vi "Test Sweep Manager.vi"(8 "error in (no error)":errorcluster, 11 "Generator in":refnum<class "Generator.lvclass">) -> (0 "error out":errorcluster, 3 "Generator out":refnum<class "Generator.lvclass">)   [LabVIEW 2019, in "Generator.lvclass"]
uses:
  Generator.lvclass
  typedefs/Sampling--Cluster.ctl
  typedefs/Sweep.Configuration--Cluster.ctl
  typedefs/Sweep.Channel--Cluster--Array.ctl
  typedefs/Sweep.Channel--Cluster.ctl
  typedefs/Sweep.Pattern--Enum.ctl
  typedefs/AO.Channel--Cluster--Array.ctl
  typedefs/AO.Channel--Cluster.ctl
  typedefs/AO.Channel.Function--Enum.ctl
  Generator.lvclass/Generator.ctl
  typedefs/Generator.Sweep Status--enum.ctl
  typedefs/Generator.Command--enum.ctl
  Waveform.Attributes/Waveform.Attributes.lvlib
panel:
  in  "AO Channels":T1=[{"Enable?"=TRUE, "Channel"=1, "Amplitude"=0.1, "Offset"=0.0, "Frequency"=13.0, "Phase"=0.0, "Function"=enum."sine", "Sweeping?"=FALSE, "Limit AC?"=FALSE, "Limit DC?"=FALSE, "Duty Cycle?"=FALSE, "Duty Cycle"=0.0}, {"Enable?"=TRUE, "Channel"=0, "Amplitude"=0.0, "Offset"=0.09, "Frequency"=0.1, "Phase"=0.0, "Function"=enum."sine", "Sweeping?"=FALSE, "Limit AC?"=FALSE, "Limit DC?"=FALSE, "Duty Cycle?"=FALSE, "Duty Cycle"=0.0}, {"Enable?"=TRUE, "Channel"=0, "Amplitude"=0.0, "Offset"=0.0, "Frequency"=0.1, "Phase"=0.0, "Function"=enum."sine", "Sweeping?"=FALSE, "Limit AC?"=FALSE, "Limit DC?"=FALSE, "Duty Cycle?"=FALSE, "Duty Cycle"=0.0}, {"Enable?"=TRUE, "Channel"=0, "Amplitude"=0.0, "Offset"=0.01, "Frequency"=0.1, "Phase"=0.0, "Function"=enum."sine", "Sweeping?"=FALSE, "Limit AC?"=FALSE, "Limit DC?"=FALSE, "Duty Cycle?"=FALSE, "Duty Cycle"=0.0}]
  out "Appended vs sample":dbl[][](graph)
  out "Concatenated":waveform(dbl)[](graph)
  out "Appended vs time":waveform(dbl)[](graph)
  in  "Sweep Pattern":cluster{"Channel":u16, "Sweep Pattern":dbl[]}[](array[cluster])=[{"Channel"=4, "Sweep Pattern"=[0.01, 0.02, 0.015, 0.025, 0.02, 0.03]}] {"Sweep Pattern" format="%#_3p"; "Channel" min=1 max=128}
  out "Updates":i32=14
  out "Live":waveform(dbl)[](graph)
  in  "Configuration.Sweep":T4={"Sweep Time (s)"=100.0, "Initial Wait (s)"=0.1, "Return to Start"=TRUE, "Channels"=[{"Enable?"=TRUE, "Channel"=1, "Start"=0.0, "End"=0.1, "Pattern"=enum."Smooth Ramp _/\\_", "Table"=[]}, {"Enable?"=TRUE, "Channel"=2, "Start"=0.09, "End"=0.09, "Pattern"=enum."Smooth Ramp _/\\_", "Table"=[]}, {"Enable?"=TRUE, "Channel"=3, "Start"=0.0, "End"=0.01, "Pattern"=enum."Ramp /\\", "Table"=[]}, {"Enable?"=TRUE, "Channel"=4, "Start"=0.01, "End"=0.011, "Pattern"=enum."Table", "Table"=[]}]} {"Channels"."Table" format="%#_1f"; "Channels"."Channel" min=1 max=128; "Channels"."Start" format="%#_6p"; "Channels"."End" format="%#_6p"}
  in  "Sampling":T8={"Fs"=10000.0, "#s"=1000.0}
  in  "stop":bool
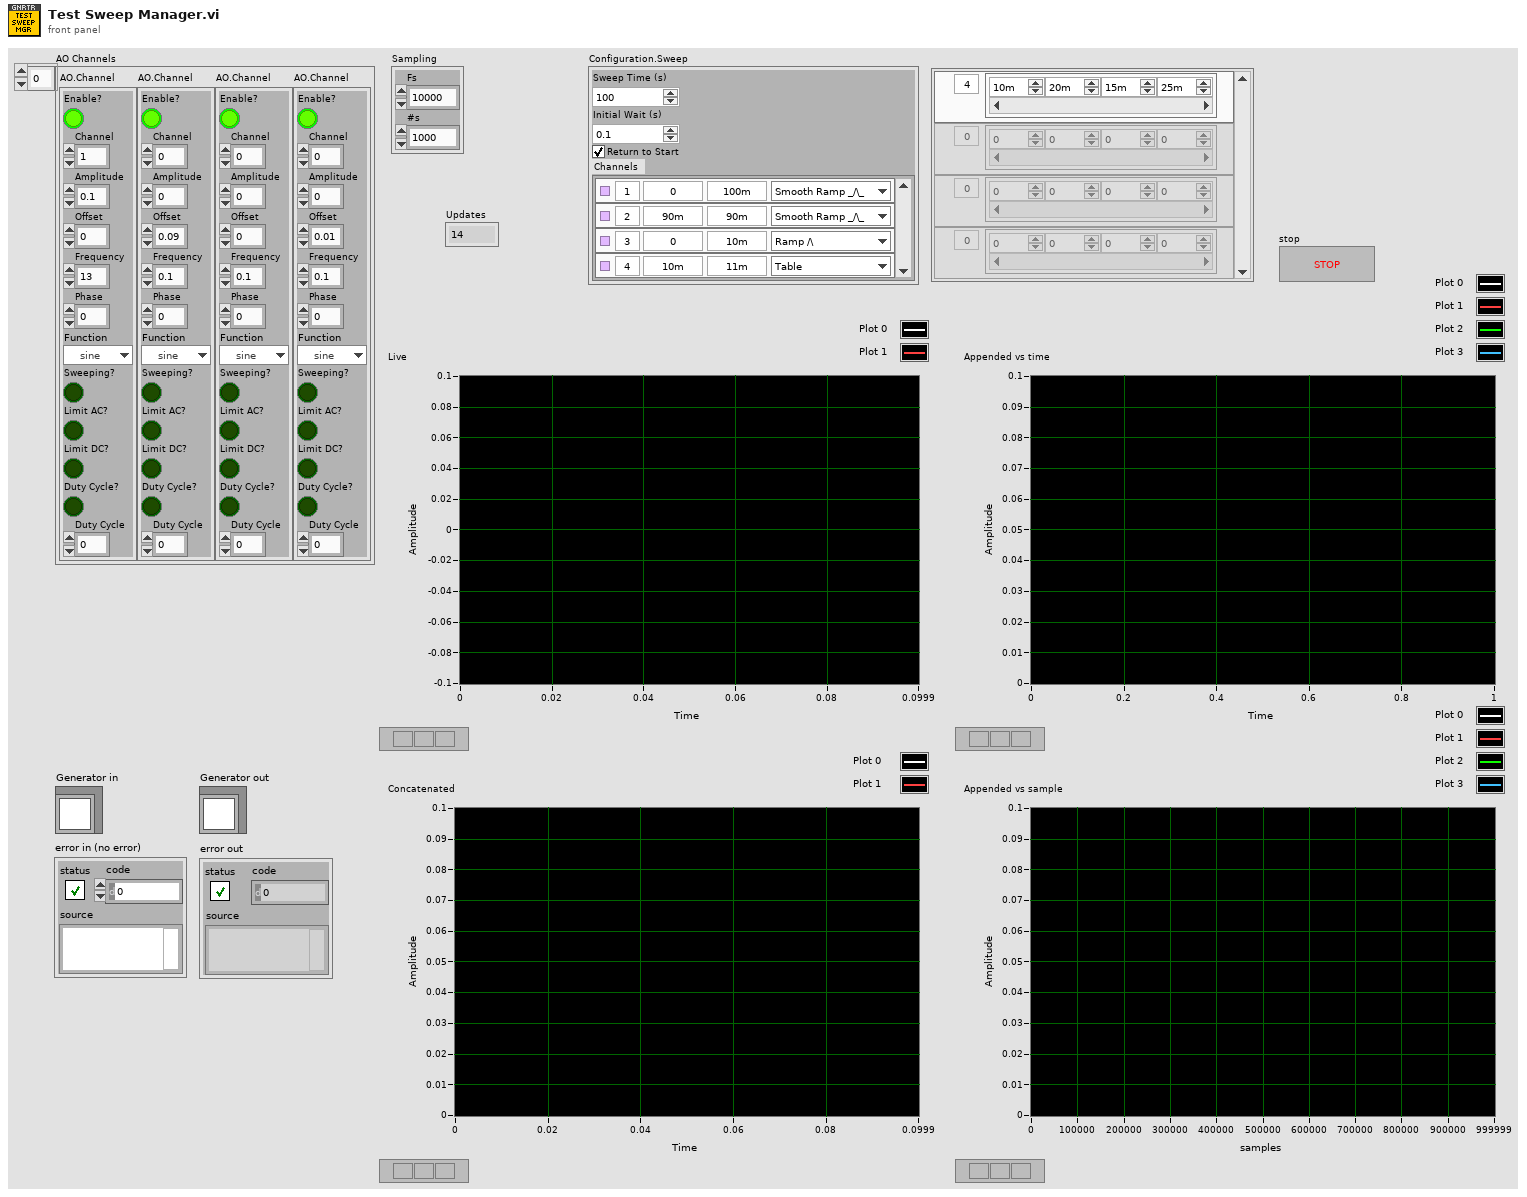
[diagram p1: front panel]
types:
  T1 = typedef "Generator.lvclass/AO.Channel--Cluster--Array.ctl" = T2[]
  T2 = typedef "Generator.lvclass/AO.Channel--Cluster.ctl" = cluster{"Enable?":bool, "Channel":i32, "Amplitude":dbl, "Offset":dbl, "Frequency":dbl, "Phase":dbl, "Function":T3, "Sweeping?":bool, "Limit AC?":bool, "Limit DC?":bool, "Duty Cycle?":bool, "Duty Cycle":dbl}
  T3 = typedef "Generator.lvclass/AO.Channel.Function--Enum.ctl" = enum16{"sine", "square", "triangle", "saw"}
  T4 = typedef "Generator.lvclass/Sweep.Configuration--Cluster.ctl" = cluster{"Sweep Time (s)":dbl, "Initial Wait (s)":dbl, "Return to Start":bool, "Channels":T5}
  T5 = typedef "Generator.lvclass/Sweep.Channel--Cluster--Array.ctl" = T6[]
  T6 = typedef "Generator.lvclass/Sweep.Channel--Cluster.ctl" = cluster{"Enable?":bool, "Channel":u16, "Start":dbl, "End":dbl, "Pattern":T7, "Table":dbl[]}
  T7 = typedef "Generator.lvclass/Sweep.Pattern--Enum.ctl" = enum16{"Ramp /", "Ramp /\\", "Smooth Ramp _/", "Smooth Ramp _/\\_", "Table"}
  T8 = typedef "Generator.lvclass/Sampling--Cluster.ctl" = cluster{"Fs":dbl, "#s":dbl}
  T9 = typedef "Generator.lvclass/Generator.Sweep Status--enum.ctl" = enum16{"idle", "initializing", "waiting", "sweeping", "stopping"}
  T10 = typedef "Generator.lvclass/Generator.Command--enum.ctl" = enum16{"start", "stop", "start sweep", "stop sweep"}
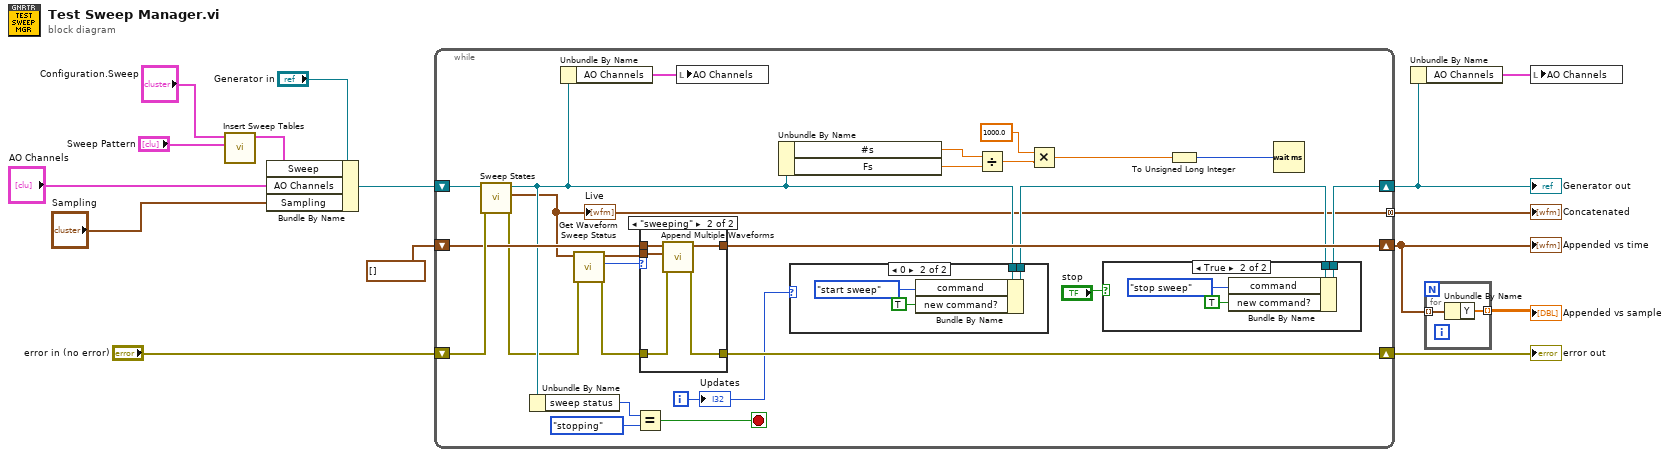
[diagram p0: block diagram]
diagram:
  n1 = call "Insert Sweep Tables.vi"("Channels New"="Sweep Pattern", "Sweep Configuration in"="Configuration.Sweep") -> ("Sweep Configuration out"=w11:T4)  [unwired: 9 in]
  n2 = Bundle By Name(cluster="Generator in", "Sweep"=w11, "AO Channels"="AO Channels", "Sampling"="Sampling") -> (w3:refnum<class "Generator.lvclass">)
  n3 = while {
    shift-right: [w39] -> w15
    shift-left: "error in (no error)" -> [w40]
    shift-right: [w35] -> w8
    shift-left: w3 -> [w36]
    shift-right: [w37] -> w2
    shift-left: waveform(dbl)[] [] ("Waveform out []") -> [w38]
    tunnel: [w20] -> w6 mode=concatenating
    i -> [w32]
    stop <- w30 stop-if-true
    n4 = call "Sweep States.vi"("error in (no error)"=w40, "Generator in"=w36) -> ("error out"=w17:errorcluster, "Waveforms out"=w20:waveform(dbl)[], "Generator out"=w29:refnum<class "Generator.lvclass">)  [unwired: 7 in]
    "Live" <- w20
    n5 = Unbundle By Name(w29) -> ("sweep status"=w21:T9)
    n6 = Unbundle By Name(w29) -> ("AO Channels"=w22:T1)
    n7 = call "Get Waveform Sweep Status.vi"("error in (no error)"=w17, "Waveforms in"=w20) -> ("error out"=w16:errorcluster, "sweep status"=w18:T9, "Waveforms out"=w19:waveform(dbl)[])  [unwired: 7 in]
    n8 = Equal?(x=w21, y=Generator.Sweep_Status--enum."stopping") -> (x = y?=w30:bool)
    n9 = case shown="\"sweeping\"" w18 {
      tunnel: [w41 w47] -> w39
      tunnel: w16 -> [w41 w46]
      tunnel: w19 -> [_ w43]
      tunnel: w38 -> [w42 w45]
      tunnel: [w42 w44] -> w37
      frame Default {
      }
      frame "sweeping" {
        n10 = call "Append Multiple Waveforms.vi"("error in (no error)"=w46, "Waveform B []"=w43, "Waveforrm A []"=w45) -> ("error out"=w47:errorcluster, "Waveform out []"=w44:waveform(dbl)[])  [unwired: 7 in]
      }
    }
    n11 = local write "AO Channels"(w22) -> ()
    n12 = Unbundle By Name(w29) -> ("#s"=w28:dbl, "Fs"=w27:dbl)
    n13 = case shown="0" w32 {
      tunnel: w29 -> [w48 w52]
      tunnel: [w48 w51] -> w33
      frame Default {
      }
      frame 0 {
        n14 = Bundle By Name(cluster=w52, "command"=Generator.Command--enum."start sweep", "new command?"=TRUE) -> (w51:refnum<class "Generator.lvclass">)
      }
    }
    n15 = Divide(x=w28, y=w27) -> (x/y=w26:dbl)
    n16 = Multiply(x=1000.0, y=w26) -> (x*y=w24:dbl)
    n17 = case shown="True" "stop" {
      tunnel: w33 -> [w53 w57]
      tunnel: [w53 w56] -> w35
      frame False {
      }
      frame True {
        n18 = Bundle By Name(cluster=w57, "command"=Generator.Command--enum."stop sweep", "new command?"=TRUE) -> (w56:refnum<class "Generator.lvclass">)
      }
    }
    n19 = To Unsigned Long Integer(number=w24) -> (unsigned 32bit integer=w23:u32)
    n20 = Wait (ms)(milliseconds to wait=w23) -> ()  [unwired: 1 out]
    "Updates" <- w32
  }
  "error out" <- w15
  "Generator out" <- w8
  "Appended vs time" <- w2
  "Concatenated" <- w6
  n21 = Unbundle By Name(w8) -> ("AO Channels"=w9:T1)
  n22 = for {
    tunnel: w2 -> [w59] mode=indexing
    tunnel: [w58] -> w1 mode=indexing
    n23 = Unbundle By Name(w59) -> ("Y"=w58:dbl[])
  }
  "Appended vs sample" <- w1
  n24 = local write "AO Channels"(w9) -> ()
